vi "initial orbit guess from individual positions.vi"(8 "error in (no error)":errorcluster, 9 "mag readings no coil":T2[](array[typedef]), 10 "crossing stats":T3, 11 "fitLocation queue":refnum<queue>) -> (0 "error out":errorcluster, 1 "ellipse parameters multi-mag":T1, 2 "mag0 ellipse parameters":T1, 3 "initial guess":T4)   [LabVIEW 2017]
uses:
  typedefs/magnet location with timestamp.ctl
  typedefs/orbit parameters full.ctl
  typedefs/crossing stats.ctl
  typedefs/magnetomter reading set.ctl
  <vilib>/Analysis/baseanly.llb/Mean (DBL).vi
  <vilib>/Analysis/NI_AALBase.lvlib
panel:
  in  "target height":dbl=55.0
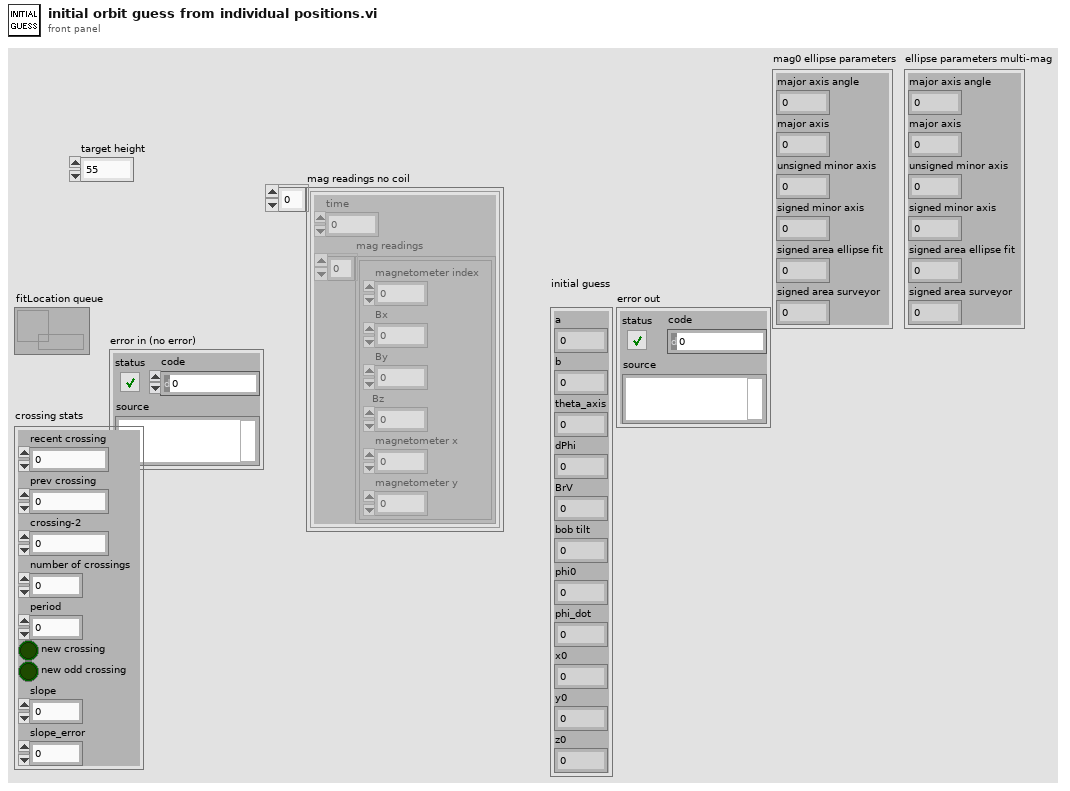
[diagram p1: front panel]
types:
  T1 = cluster{"major axis angle":dbl, "major axis":dbl, "unsigned minor axis":dbl, "signed minor axis":dbl, "signed area ellipse fit":dbl, "signed area surveyor":dbl}
  T2 = typedef "magnetomter reading set.ctl" = cluster{"time":fxp<+,48,48>, "mag readings":cluster{"magnetometer index":dbl, "Bx":dbl, "By":dbl, "Bz":dbl, "magnetometer x":dbl, "magnetometer y":dbl}[]}
  T3 = typedef "crossing stats.ctl" = cluster{"recent crossing":dbl, "prev crossing":dbl, "crossing-2":dbl, "number of crossings":i32, "period":dbl, "new crossing":bool, "new odd crossing":bool, "slope":dbl, "slope_error":dbl}
  T4 = typedef "orbit parameters full.ctl" = cluster{"a":dbl, "b":dbl, "theta_axis":dbl, "dPhi":dbl, "BrV":dbl, "bob tilt":dbl, "phi0":dbl, "phi_dot":dbl, "x0":dbl, "y0":dbl, "z0":dbl}
  T5 = typedef "magnet location with timestamp.ctl" = cluster{"x magnet":dbl, "y magnet":dbl, "z magnet":dbl, "Br*V (T*mm^3)":dbl, "theta - moment angle to z-axis":dbl, "phi - moment angle to x-axis":dbl, "measurement time":dbl}
  T6 = cluster{"magnetometer index":dbl, "Bx":dbl, "By":dbl, "Bz":dbl, "magnetometer x":dbl, "magnetometer y":dbl}[]
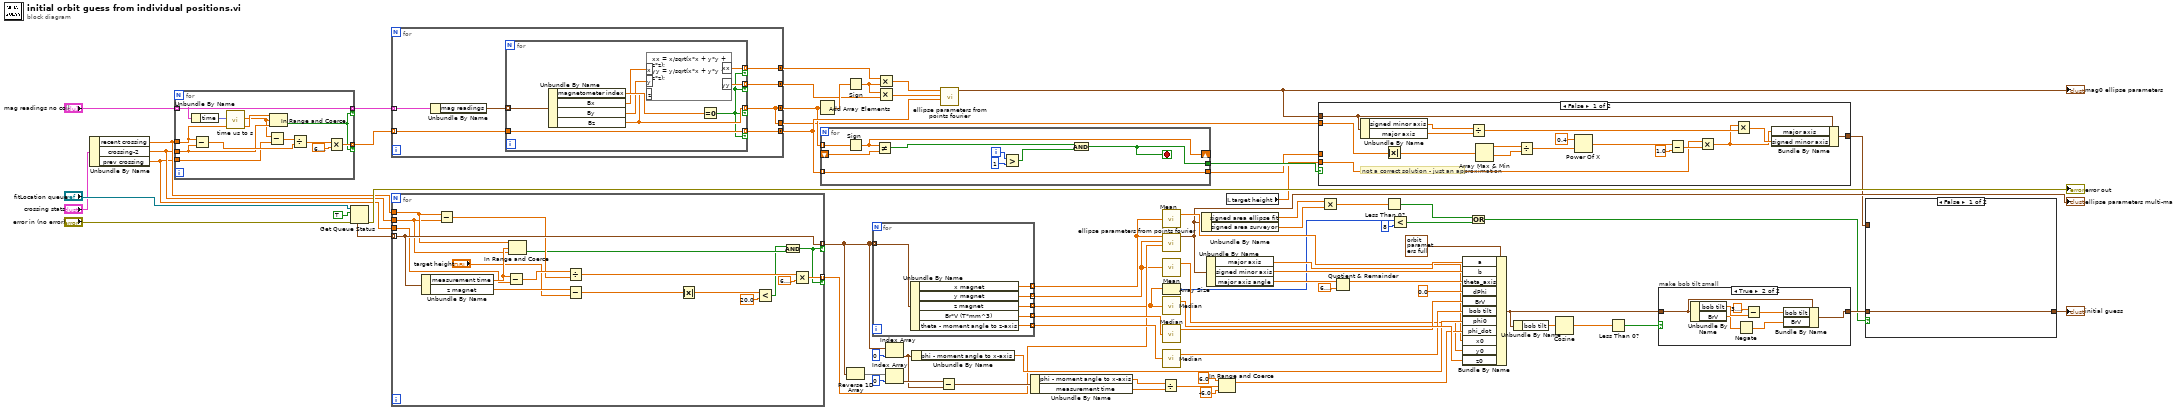
[diagram p0: block diagram]
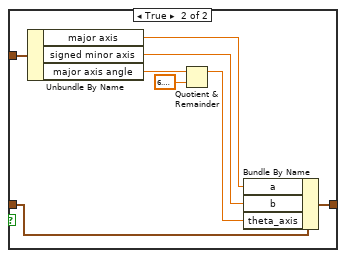
[diagram p2: hidden frame]
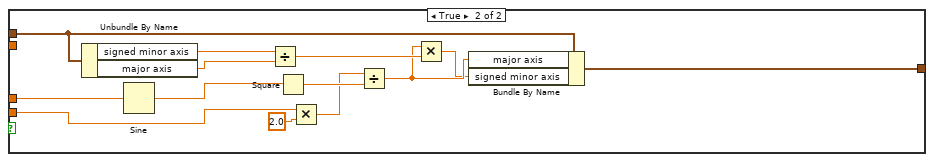
[diagram p3: hidden frame]
diagram:
  n1 = Unbundle By Name("crossing stats") -> ("recent crossing"=w40:dbl, "crossing-2"=w39:dbl, "prev crossing"=w38:dbl)
  n2 = for {
    tunnel: "mag readings no coil" -> [w85] mode=indexing
    tunnel: [w85] -> w37 mode=indexing if=w79
    tunnel: [w80] -> w36 mode=indexing if=w79
    tunnel: w40 -> [w78]
    tunnel: w39 -> [w77]
    tunnel: w38 -> [w76]
    n3 = Unbundle By Name(w85) -> ("time"=w75:fxp<+,48,48>)
    n4 = Subtract(x=w78, y=w77) -> (x-y=w83:dbl)
    n5 = call "time us to s.vi"("time (us)"=w75) -> ("time (s)"=w74:dbl)  [unwired: 10 in]
    n6 = Subtract(x=w74, y=w76) -> (x-y=w84:dbl)
    n7 = In Range and Coerce(upper limit=w78, x=w74, lower limit=w77) -> (In Range?=w79:bool)  [unwired: 1 out]
    n8 = Divide(x=w84, y=w83) -> (x/y=w82:dbl)
    n9 = Multiply(x=w82, y=6.283185307179586) -> (x*y=w80:dbl)
  }
  n10 = Get Queue Status(queue="fitLocation queue", return elements? (F)=TRUE, error in (no error)="error in (no error)") -> (error out=→"error out":errorcluster, elements=w71:T5[])  [unwired: 6 out]
  n11 = for {
    tunnel: w37 -> [w92] mode=indexing
    tunnel: [w90] -> w33 mode=concatenating
    tunnel: [w89] -> w30 mode=concatenating
    tunnel: w36 -> [w88] mode=indexing
    tunnel: [w87] -> w20 mode=concatenating
    tunnel: [w86] -> w16 mode=concatenating
    tunnel: [w86] -> w15
    n12 = Unbundle By Name(w92) -> ("mag readings"=w91:T6)
    n13 = for {
      tunnel: w91 -> [w101] mode=indexing
      tunnel: [w97] -> w90 mode=indexing if=w93
      tunnel: [w96] -> w89 mode=indexing if=w93
      tunnel: w88 -> [w95]
      tunnel: [w95] -> w87 mode=indexing if=w93
      tunnel: [w94] -> w86 mode=indexing if=w93
      n14 = Unbundle By Name(w101) -> ("magnetometer index"=w100:dbl, "Bx"=w99:dbl, "By"=w98:dbl, "Bz"=w94:dbl)
      n15 = formula code="xx = x/sqrt(x*x + y*y + z*z);\nyy = y/sqrt(x*x + y*y + z*z);"("x"=w99, "y"=w98, "z"=w94) -> ("xx"=w97:dbl, "yy"=w96:dbl)
      n16 = Equal To 0?(x=w100) -> (x = 0?=w93:bool)
    }
  }
  n17 = for {
    tunnel: w71 -> [w119] mode=indexing
    tunnel: [w119] -> w60 mode=indexing if=w103
    tunnel: [w113] -> w35 mode=indexing if=w103
    tunnel: w40 -> [w111]
    tunnel: w39 -> [w110]
    tunnel: w38 -> [w109]
    n18 = Unbundle By Name(w119) -> ("measurement time"=w118:dbl, "z magnet"=w108:dbl)
    n19 = Subtract(x=w111, y=w110) -> (x-y=w116:dbl)
    n20 = Subtract(x=w118, y=w109) -> (x-y=w117:dbl)
    n21 = In Range and Coerce(upper limit=w111, x=w118, lower limit=w110) -> (In Range?=w112:bool)  [unwired: 1 out]
    n22 = Divide(x=w117, y=w116) -> (x/y=w115:dbl)
    n23 = Subtract(x=w108, y="target height") -> (x-y=w106:dbl)
    n24 = Absolute Value(x=w106) -> (abs(x)=w105:dbl)
    n25 = Less?(x=w105, y=20.0) -> (x < y?=w102:bool)
    n26 = And(x=w102, y=w112) -> (x .and. y?=w103:bool)
    n27 = Multiply(x=w115, y=6.283185307179586) -> (x*y=w113:dbl)
  }
  n28 = Add Array Elements(numeric array=w16) -> (sum=w34:dbl)
  n29 = for {
    tunnel: w16 -> [w128] mode=indexing
    tunnel: w20 -> [w121] mode=indexing
    shift-right: [w127] -> _
    shift-left: _ -> [w126]
    tunnel: [w121] -> w18
    tunnel: [w120] -> w19
    i -> [w125]
    stop <- w120 stop-if-true
    n30 = Sign(1:w128) -> (0:w127:dbl)
    n31 = Not Equal?(x=w127, y=w126) -> (x != y?=w122:bool)
    n32 = Greater?(x=w125, y=1) -> (0:w123:bool)
    n33 = And(x=w122, y=w123) -> (x .and. y?=w120:bool)
  }
  n34 = Sign(1:w34) -> (0:w31:dbl)
  n35 = Reverse 1D Array(array=w60) -> (reversed array=w59:T5[])
  n36 = for {
    tunnel: w60 -> [w134] mode=indexing
    tunnel: [w133] -> w24 mode=indexing
    tunnel: [w132] -> w23 mode=indexing
    tunnel: [w131] -> w7 mode=indexing
    tunnel: [w130] -> w70 mode=indexing
    tunnel: [w129] -> w64 mode=indexing
    n37 = Unbundle By Name(w134) -> ("x magnet"=w133:dbl, "y magnet"=w132:dbl, "z magnet"=w131:dbl, "Br*V (T*mm^3)"=w130:dbl, "theta - moment angle to z-axis"=w129:dbl)
  }
  n38 = Multiply(x=w33, y=w31) -> (x*y=w32:dbl[])
  n39 = Multiply(x=w31, y=w30) -> (x*y=w29:dbl[])
  n40 = Index Array(array=w60, index=0) -> (element=w56:T5)
  n41 = Index Array(array=w59, index=0) -> (element=w57:T5)
  n42 = Unbundle By Name(w56) -> ("phi - moment angle to x-axis"=w61:dbl)
  n43 = Subtract(x=w57, y=w56) -> (x-y=w55:T5)
  n44 = call "ellipse parameters from points fourier.vi"("Phi"=w20, "Y"=w29, "X"=w32) -> ("ellipse parameters"=w17:T1)  [unwired: 8 in]
  "mag0 ellipse parameters" <- w17
  n45 = Unbundle By Name(w55) -> ("phi - moment angle to x-axis"=w54:dbl, "measurement time"=w53:dbl)
  n46 = Divide(x=w54, y=w53) -> (x/y=w52:dbl)
  n47 = call-poly <vilib>:"Mean.vi"("X"=w24) -> ("mean"=w22:dbl)  [unwired: 1 out]
  n48 = call "ellipse parameters from points fourier.vi"("Phi"=w35, "Y"=w23, "X"=w24) -> ("ellipse parameters"=w13:T1)  [unwired: 8 in]
  "ellipse parameters multi-mag" <- w13
  n49 = call-poly <vilib>:"Mean.vi"("X"=w23) -> ("mean"=w21:dbl)  [unwired: 1 out]
  n50 = Array Size(array=w7) -> (size(s)=w6:i32)
  n51 = call <vilib>:"Median.vi"("X"=w7) -> ("median"=w67:dbl)  [unwired: 1 out]
  n52 = call <vilib>:"Median.vi"("X"=w70) -> ("median"=w66:dbl)  [unwired: 1 out]
  n53 = call <vilib>:"Median.vi"("X"=w64) -> ("median"=w63:dbl)  [unwired: 1 out]
  n54 = Unbundle By Name(w13) -> ("signed area ellipse fit"=w12:dbl, "signed area surveyor"=w11:dbl)
  n55 = Unbundle By Name(w13) -> ("major axis"=w28:dbl, "signed minor axis"=w27:dbl, "major axis angle"=w26:dbl)
  n56 = In Range and Coerce(upper limit=6.0, x=w52, lower limit=-6.0) -> (coerced(x)=w49:dbl)  [unwired: 1 out]
  n57 = local read "target height"() -> (w14:dbl)
  n58 = case shown="False" w19 {
    tunnel: w18 -> [_ w164]
    tunnel: w17 -> [w137 w156]
    tunnel: [w135 w153] -> w2
    tunnel: w15 -> [w150 _]
    tunnel: w14 -> [w142 w152]
    frame False {
      # "not a correct solution - just an approximation"
      n59 = Unbundle By Name(w137) -> ("signed minor axis"=w141:dbl, "major axis"=w140:dbl)
      n60 = Absolute Value(x=w150) -> (abs(x)=w151:dbl[])
      n61 = Divide(x=w141, y=w140) -> (x/y=w139:dbl)
      n62 = Array Max & Min(array=w151) -> (max value=w149:dbl, min value=w148:dbl)  [unwired: 2 out]
      n63 = Divide(x=w149, y=w148) -> (x/y=w147:dbl)
      n64 = Power Of X(1:w147, 2:0.4 ("y")) -> (0:w145:dbl)
      n65 = Subtract(x=w145, y=1.0) -> (x-y=w143:dbl)
      n66 = Multiply(x=w142, y=w143) -> (x*y=w136:dbl)
      n67 = Multiply(x=w136, y=w139) -> (x*y=w138:dbl)
      n68 = Bundle By Name(cluster=w137, "major axis"=w136, "signed minor axis"=w138) -> (w135:T1)
    }
    frame True {
      n69 = Unbundle By Name(w156) -> ("signed minor axis"=w161:dbl, "major axis"=w160:dbl)
      n70 = Sine(x=w164) -> (sin(x)=w163:dbl)
      n71 = Divide(x=w161, y=w160) -> (x/y=w159:dbl)
      n72 = Square(x=w163) -> (x^2=w162:dbl)
      n73 = Multiply(x=w152, y=2.0) -> (x*y=w158:dbl)
      n74 = Divide(x=w158, y=w162) -> (x/y=w155:dbl)
      n75 = Multiply(x=w155, y=w159) -> (x*y=w154:dbl)
      n76 = Bundle By Name(cluster=w156, "major axis"=w155, "signed minor axis"=w154) -> (w153:T1)
    }
  }
  n77 = Multiply(x=w12, y=w11) -> (x*y=w10:dbl)
  n78 = Quotient & Remainder(x=w26, y=6.283185307179586) -> (x-y*floor(x/y)=w25:dbl)  [unwired: 1 out]
  n79 = Less Than 0?(x=w10) -> (x < 0?=w8:bool)
  n80 = Less?(x=w6, y=8) -> (x < y?=w3:bool)
  n81 = Bundle By Name(cluster=T4 {"a"=0.0, "b"=0.0, "theta_axis"=0.0, "dPhi"=0.0, "BrV"=0.0, "bob tilt"=0.0, "phi0"=0.0, "phi_dot"=0.0, "x0"=0.0, "y0"=0.0, "z0"=0.0} ("orbit parameters"), "a"=w28, "b"=w27, "theta_axis"=w25, "dPhi"=0.0, "BrV"=w66, "bob tilt"=w63, "phi0"=w61, "phi_dot"=w49, "x0"=w22, "y0"=w21, "z0"=w67) -> (w43:T4)
  n82 = Or(x=w8, y=w3) -> (x .or. y?=w4:bool)
  n83 = Unbundle By Name(w43) -> ("bob tilt"=w46:dbl)
  n84 = Cosine(x=w46) -> (cos(x)=w45:dbl)
  n85 = Less Than 0?(x=w45) -> (x < 0?=w44:bool)
  n86 = case "make bob tilt small" shown="True" w44 {
    tunnel: w43 -> [w165 w170]
    tunnel: [w165 w167] -> w9
    frame False {
    }
    frame True {
      n87 = Unbundle By Name(w170) -> ("bob tilt"=w171:dbl, "BrV"=w169:dbl)
      n88 = Negate(x=w169) -> (-x=w168:dbl)
      n89 = Subtract(x=3.141592653589793, y=w171) -> (x-y=w166:dbl)
      n90 = Bundle By Name(cluster=w170, "bob tilt"=w166, "BrV"=w168) -> (w167:T4)
    }
  }
  n91 = case shown="False" w4 {
    tunnel: w9 -> [w173 w181]
    tunnel: w2 -> [_ w180]
    tunnel: [w173 w174] -> w1
    frame False {
    }
    frame True {
      n92 = Unbundle By Name(w180) -> ("major axis"=w178:dbl, "signed minor axis"=w179:dbl, "major axis angle"=w176:dbl)
      n93 = Quotient & Remainder(x=w176, y=6.283185307179586) -> (x-y*floor(x/y)=w175:dbl)  [unwired: 1 out]
      n94 = Bundle By Name(cluster=w181, "a"=w178, "b"=w179, "theta_axis"=w175) -> (w174:T4)
    }
  }
  "initial guess" <- w1
